vi "Destroy.vi"(8 "Error In":errorcluster, 11 "Communicator in":refnum<class "Communicator.lvclass">) -> (0 "Error Out":errorcluster, 3 "Communicator out":refnum<class "Communicator.lvclass">)   [LabVIEW 2024, in "Communicator.lvclass"]
uses:
  Communicator.lvclass
  Source/Interfaces/IInstrument/IInstrument.lvclass
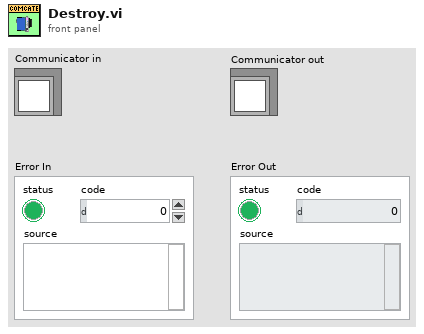
[diagram p1: front panel]
types:
  T1 = typedef "Communicator.lvclass/ObjectAttributes.ctl" = cluster{"IConfigure":refnum<class "IConfigure.lvclass">}
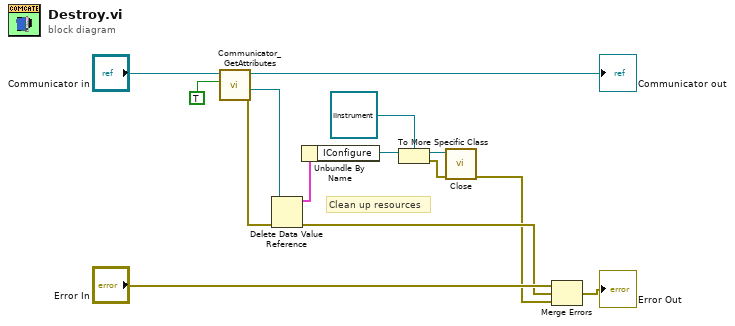
[diagram p0: block diagram]
diagram:
  # "Clean up resources"
  n1 = call "Communicator_GetAttributes.vi"("OnlyGetDvrReference(False)"=TRUE, "Communicator in"="Communicator in") -> ("Error Out"=w11:errorcluster, "DataRef"=w10:refnum<data-value>, "Communicator out"=→"Communicator out":refnum<class "Communicator.lvclass">)  [unwired: 6 in, 1 out]
  n2 = Delete Data Value Reference(data value reference=w10, error in=w11) -> (data value=w7:T1, error out=w2:errorcluster)
  n3 = Unbundle By Name(w7) -> ("IConfigure"=w6:refnum<class "IConfigure.lvclass">)
  n4 = To More Specific Class(target class=refnum<class "IInstrument.lvclass"> refnum ("IInstrument.lvclass"), reference=w6) -> (specific class reference=w3:refnum<class "IInstrument.lvclass">, error out=w4:errorcluster)  [unwired: 1 in]
  n5 = call-dynamic "Close.vi"("error in"=w4, "IInstrument in"=w3) -> ("error out"=w1:errorcluster)  [unwired: 8 in, 1 out]
  n6 = Merge Errors("Error In", w2, w1) -> (→"Error Out":errorcluster)
